vi "find min power for drive.vi"(10 "distance":dbl) -> (0 "Min power":dbl)   [LabVIEW 2017]
uses:
  <vilib>/Rock Robotics/WPI/Utilities/WPI_GetSetVariantRefNum.vi
  <vilib>/Rock Robotics/WPI/RobotDrive/WPI_RobotDriveArcadeDrive_Standard(NoSaturation).vi
panel:
  out "running?":bool
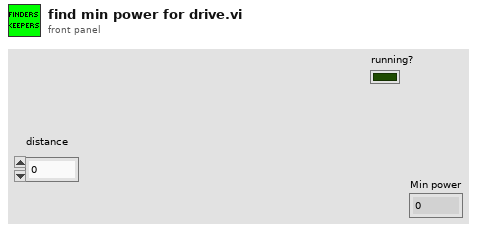
[diagram p1: front panel]
types:
  T1 = typedef "WPI_EncoderDevRef.ctl" = cluster{"DevStatus":errorcluster, "EncoderIndex":T2, "CounterIndex":T3, "DistancePerCount":dbl, "Decoding Type":T4}
  T2 = typedef "FPGA_EncoderIdx.ctl" = enum8{"Enc 0", "Enc 1", "Enc 2", "Enc 3", "Enc 4", "Enc 5", "Enc 6", "Enc 7", "Invalid"}
  T3 = typedef "FPGA_CounterCtrSystemIndex.ctl" = enum8{"Ctr 0", "Ctr 1", "Ctr 2", "Ctr 3", "Ctr 4", "Ctr 5", "Ctr 6", "Ctr 7", "Invalid"}
  T4 = typedef "WPI_EncoderType.ctl" = enum16{"1x", "2x", "4x"}
  T5 = typedef "WPI_RobotDriveDevRef.ctl" = cluster{"DevStatus":errorcluster, "Motors[]":T6[], "Square Inputs":bool, "Max Output":dbl}
  T6 = typedef "WPI_MotorControlDeviceRef.ctl" = cluster{"DeviceStatus":errorcluster, "Type":T7, "PWM":cluster{"PWM Channel":T8, "DeadBand":T9}, "CAN":cluster{"Device Number":u8, "SetOutput VI Ref":variant, "GetOutput VI Ref":variant, "Enable VI Ref":variant, "Disable VI Ref":variant, "Data":variant}, "Invert":bool, "DIO PWM":cluster{"PWM \"Enable\" Channel":T8, "DIOChannel":T10, "PWM Rate":dbl}}
  T7 = typedef "WPI_MotorControlType.ctl" = enum16{"PWM", "CAN", "DIO PWM"}
  T8 = typedef "FPGA_DIOPWMChannel.ctl" = enum8{"PWM 0", "PWM 1", "PWM 2", "PWM 3", "PWM 4", "PWM 5", "PWM 6", "PWM 7", "PWM 8", "PWM 9", "PWM MXP 0", "PWM MXP 1", "PWM MXP 2", "PWM MXP 3", "PWM MXP 4", "PWM MXP 5", "PWM MXP 6", "PWM MXP 7", "PWM MXP 8", "PWM MXP 9", "Invalid"}
  T9 = typedef "WPI_PWMDeadband.ctl" = cluster{"Name":string, "maxPositivePwm":i32, "minPositivePwm":i32, "centerPwm":i32, "maxNegativePwm":i32, "minNegativePwm":i32, "angularRange":u16}
  T10 = typedef "FPGA_DIOChannel.ctl" = enum8{"DIO 0", "DIO 1", "DIO 2", "DIO 3", "DIO 4", "DIO 5", "DIO 6", "DIO 7", "DIO 8", "DIO 9", "DIO MXP 0", "DIO MXP 1", "DIO MXP 2", "DIO MXP 3", "DIO MXP 4", "DIO MXP 5", "DIO MXP 6", "DIO MXP 7", "DIO MXP 8", "DIO MXP 9", "DIO MXP 10", "DIO MXP 11", "DIO MXP 12", "DIO MXP 13", "DIO MXP 14", "DIO MXP 15", "SPI Port CS1", "SPI Port CS2", "SPI Port CS3", "SPI Port MISO", "SPI Port MOSI", "Invalid"}
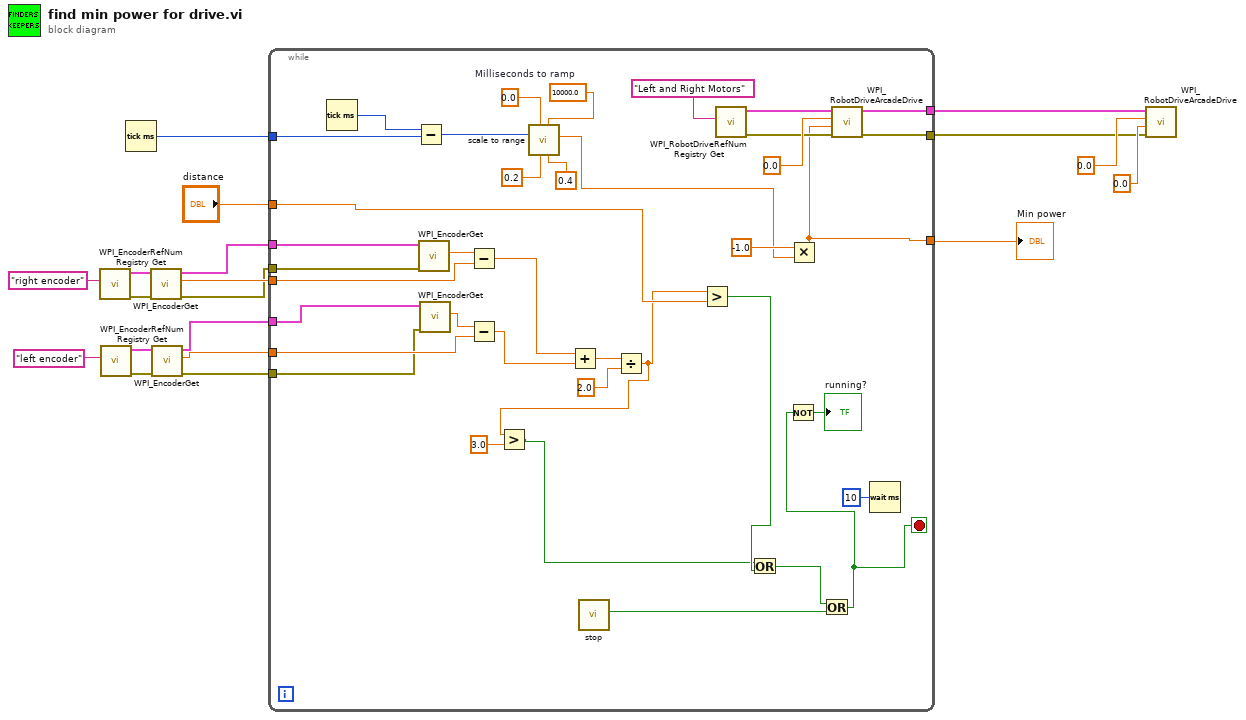
[diagram p0: block diagram]
diagram:
  n1 = call <vilib>:"WPI_EncoderRefNum Registry Get.vi"("refnum name"="right encoder") -> ("error out"=w19:errorcluster, "EncoderDevRef"=w18:T1)  [unwired: 9 in]
  n2 = call <vilib>:"WPI_EncoderRefNum Registry Get.vi"("refnum name"="left encoder") -> ("error out"=w16:errorcluster, "EncoderDevRef"=w15:T1)  [unwired: 9 in]
  n3 = Tick Count (ms)() -> (millisecond timer value=w3:u32)
  n4 = call <vilib>:"WPI_EncoderGet.vi"("error in (no error)"=w19, "EncoderDevRef"=w18) -> ("error out"=w6:errorcluster, "Distance"=w13:dbl, "EncoderDevRef"=w7:T1)  [unwired: 4 in, 3 out]
  n5 = call <vilib>:"WPI_EncoderGet.vi"("error in (no error)"=w16, "EncoderDevRef"=w15) -> ("error out"=w5:errorcluster, "Distance"=w12:dbl, "EncoderDevRef"=w4:T1)  [unwired: 4 in, 3 out]
  n6 = while {
    tunnel: "distance" -> [w40]
    tunnel: w13 -> [w50]
    tunnel: w12 -> [w51]
    tunnel: [w49] -> w9
    tunnel: [w48] -> w8
    tunnel: w7 -> [w47]
    tunnel: w6 -> [w46]
    tunnel: w5 -> [w45]
    tunnel: w4 -> [w44]
    tunnel: w3 -> [w37]
    tunnel: [w25] -> w2
    stop <- w21 stop-if-true
    w34 = 10000.0  # Milliseconds to ramp
    n7 = Tick Count (ms)() -> (millisecond timer value=w36:u32)
    n8 = Subtract(x=w36, y=w37) -> (x-y=w31:u32)
    n9 = call <vilib>:"WPI_EncoderGet.vi"("error in (no error)"=w46, "EncoderDevRef"=w47) -> ("Distance"=w53:dbl)  [unwired: 4 in, 5 out]
    n10 = call <vilib>:"WPI_EncoderGet.vi"("error in (no error)"=w45, "EncoderDevRef"=w44) -> ("Distance"=w52:dbl)  [unwired: 4 in, 5 out]
    n11 = Subtract(x=w53, y=w50) -> (x-y=w41:dbl)
    n12 = Subtract(x=w52, y=w51) -> (x-y=w30:dbl)
    n13 = call "scale to range.vi"("Max"=0.4 ("Min"), "High"=w34, "Min"=0.2, "Low"=0.0, "In Signal"=w31) -> ("Output signal"=w24:dbl)  [unwired: 6 in]
    n14 = Add(x=w41, y=w30) -> (x+y=w43:dbl)
    n15 = call "stop.vi"() -> ("Boolean"=w22:bool)  [unwired: 11 in]
    n16 = Divide(x=w43, y=2.0) -> (x/y=w27:dbl)
    n17 = Greater?(x=w27, y=3.0) -> (0:w28:bool)
    n18 = Greater?(x=w27, y=w40) -> (0:w29:bool)
    n19 = call <vilib>:"WPI_RobotDriveRefNum Registry Get.vi"("refnum name"="Left and Right Motors") -> ("error out"=w55:errorcluster, "RobotDriveDevRef"=w54:T5)  [unwired: 1 in, 8 out]
    n20 = Or(x=w28, y=w29) -> (x .or. y?=w20:bool)
    n21 = Multiply(x=-1.0, y=w24) -> (x*y=w25:dbl)
    n22 = Or(x=w20, y=w22) -> (x .or. y?=w21:bool)
    n23 = Not(x=w21) -> (.not. x?=→"running?":bool)
    n24 = call-poly <vilib>:"WPI_RobotDriveArcadeDrive.vi"("error in (no error)"=w55, "Y axis value"=w25, "X axis value"=0.0, "RobotDriveDevRef"=w54) -> ("error out"=w49:errorcluster, "RobotDriveDevRef"=w48:T5)  [unwired: 6 out]
    n25 = Wait (ms)(milliseconds to wait=u32 10) -> ()  [unwired: 1 out]
  }
  "Min power" <- w2
  n26 = call-poly <vilib>:"WPI_RobotDriveArcadeDrive.vi"("error in (no error)"=w9, "Y axis value"=0.0 ("X axis value"), "X axis value"=0.0, "RobotDriveDevRef"=w8) -> ()  [unwired: 8 out]
